vi "StepperServoMotors.vi"() -> ()   [LabVIEW 2016]
uses:
  VIs/uPythonX/uPythonX.xctl
panel:
  in  "Servo":T1(xcontrol)={"VISA Refnum in"="ASRL42::INSTR", "All Code"="'''\nhttps://docs.micropython.org/en/latest/pyboard/tutorial/servo.html\n     \nconnections: \nGround (B) - GND \nPower  (R)   - 3V3 \nNC\nSignal -  pin X1\n'''\n\nimport pyb\n\nservo1 = pyb.Servo(1)   # pix X1\n\n#set the angle\nservo1.angle(45)\n\n#read the angle\nservo1.angle()\n\n# move two servos at the same time with speed control\nservo2 = pyb.Servo(2)   \nservo1.angle(-45, 2000); servo2.angle(60, 2000)\n\n# continuous rotation\nservo1.speed()\n\n# you can also change the calibration (see webpage)\n\n"}
  in  "Stepper":T1(xcontrol)={"VISA Refnum in"="ASRL42::INSTR", "All Code"="'''\nhttps://www.amazon.com/ELEGOO-28BYJ-48-ULN2003-Stepper-Arduino/dp/B01CP18J4A?ref_=fsclp_pl_dp_2     \n\nconnections: \nGround (B) - GND \nPower  (R)   - separate 5v power supply \nIN1 = W29\nIN2 = W24\nIN3 = W22\nIN4 = W16\n'''\n\nfrom pyb import Pin\nimport utime\n\nsequence = [(0,0,0,1),(0,0,1,1),(0,0,1,0),(0,1,1,0),\n                    (0,1,0,0),(1,1,0,0),(1,0,0,0),(1,0,0,1)]\n\n\nIN1 = Pin('W29',Pin.OUT)\nIN2 = Pin('W24',Pin.OUT)\nIN3 = Pin('W22',Pin.OUT)\nIN4 = Pin('W16',Pin.OUT)\n\ndef stepper(Steps,Direction):\n     steps = 0\n     for i in range(Steps):\n#          print(str(steps) + ' : ' + str(sequence[steps]))\n          utime.sleep_us(800)\n          IN1.value(sequence[steps][0])\n          IN2.value(sequence[steps][1])\n          IN3.value(sequence[steps][2])\n          IN4.value(sequence[steps][3])\n          if Direction:\n               steps += 1\n          else:\n               steps -= 1\n          if steps < 0:\n               steps = 7\n          elif steps > 7:\n               steps = 0\n     return Steps\n\n\nfor i in range(10):\n     rotations = 1.5\n     steps = int(rotations * 4096)\n     stepper(steps,True)\n     utime.sleep(1)\n\n\n\n\n\n\n\n\n\n\n\n\n\n\n\n\n\n"}
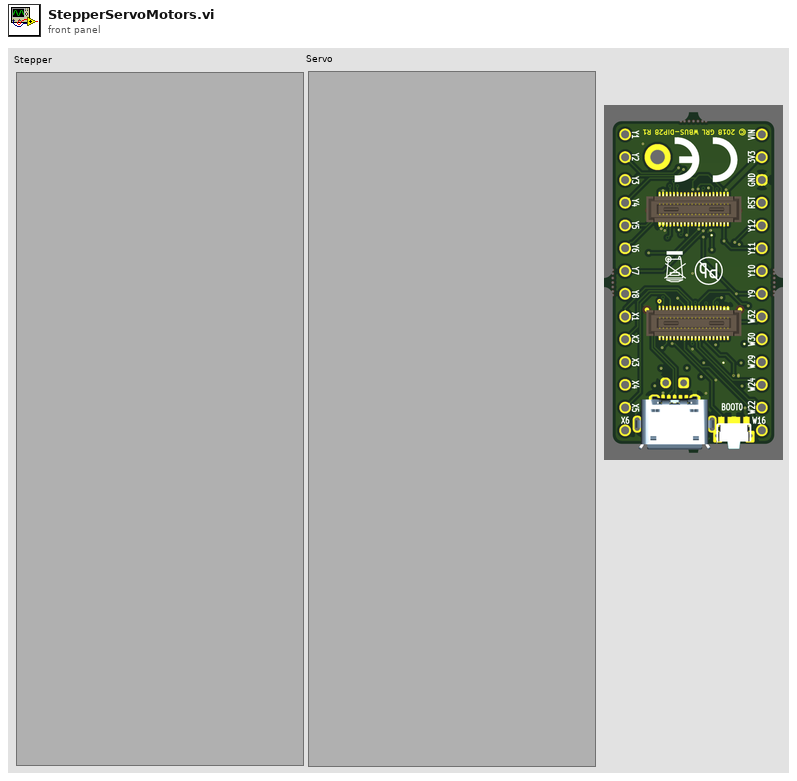
[diagram p1: front panel]
types:
  T1 = cluster{"VISA Refnum in":refnum<visa-resource-name>, "All Code":string}
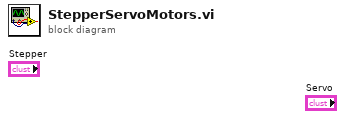
[diagram p0: block diagram]
diagram:
